vi "encodeStream.vi"(8 "error in (no error)":errorcluster, 11 "tBSONJavaScriptWithScope in":refnum<class "tBSONJavaScriptWithScope.lvclass">) -> (0 "error out":errorcluster, 2 "Byte Array":u8[](array[numeric]), 3 "tBSONJavaScriptWithScope out":refnum<class "tBSONJavaScriptWithScope.lvclass">)   [LabVIEW 2013, in "BSON.lvlib" / "tBSONJavaScriptWithScope.lvclass"]
uses:
  tBSONJavaScriptWithScope.lvclass
  tBSONElement/getName.vi
  tBSONJavaScript/getScript.vi
  getScope.vi
  tBSONDocument/tBSONDocument.lvclass
  BSON.lvlib
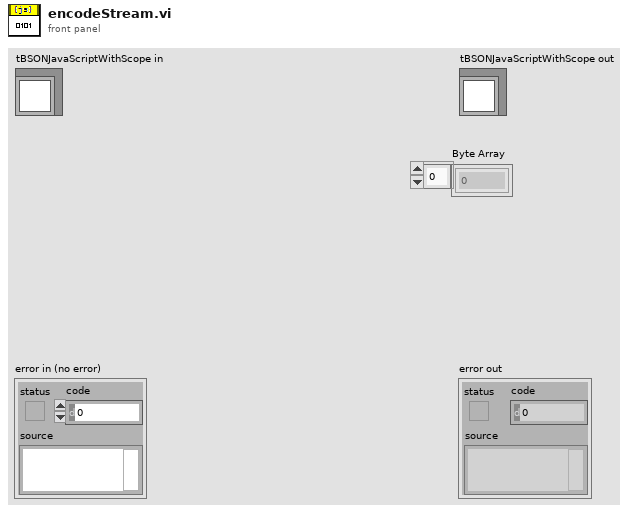
[diagram p1: front panel]
types:
  T1 = typedef "BSON.lvlib/tBSONElement.lvclass/type.ctl" = u8
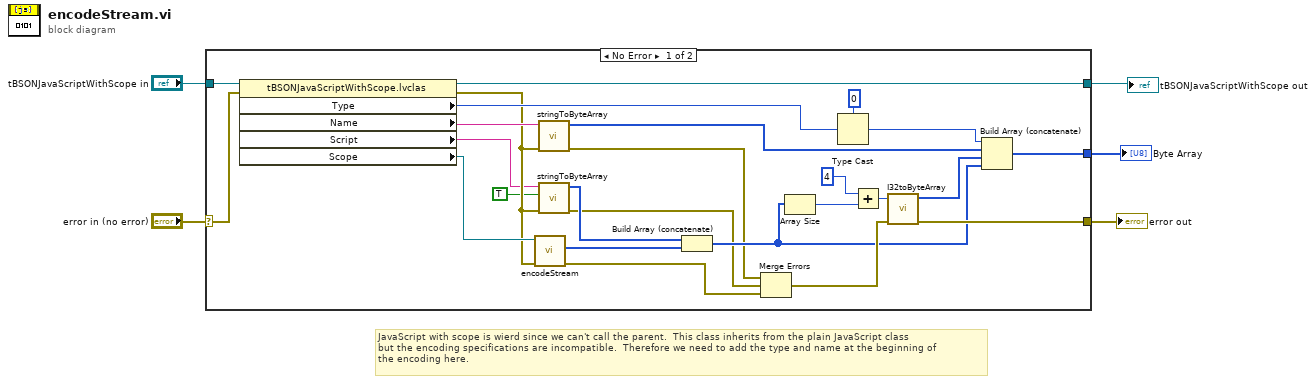
[diagram p0: block diagram]
diagram:
  # "JavaScript with scope is wierd since we can't call the parent.  This class inherits from the plain JavaScript class\nbut the encoding specifications are incompatible.  Therefore we need to add the type and name at the beginning of\nthe encoding here."
  n1 = case shown="No Error" "error in (no error)" {
    selector: "error in (no error)" -> [w29 w31]
    tunnel: "tBSONJavaScriptWithScope in" -> [w30 w32]
    tunnel: [w17 w32] -> w1
    tunnel: [w21 w31] -> w3
    tunnel: [w28 _] -> w2
    frame No Error {
      n2 = property class="tBSONJavaScriptWithScope.lvclas"(reference=w30, error in=w29) -> (reference out=w17:refnum<class "tBSONJavaScriptWithScope.lvclass">, error out=w10:errorcluster, "Type"=w15:T1, "Name"=w13:string, "Script"=w9:string, "Scope"=w26:refnum<class "tBSONDocument.lvclass">)
      n3 = call "encodeStream.vi"("error in (no error)"=w10, "tBSONDocument in"=w26) -> ("error out"=w27:errorcluster, "Byte Data"=w20:u8[])  [unwired: 7 in, 1 out]
      n4 = call "stringToByteArray.vi"("error in (no error)"=w10, "String"=w13) -> ("error out"=w12:errorcluster, "byte array"=w11:u8[])  [unwired: 8 in]
      n5 = call "stringToByteArray.vi"("error in (no error)"=w10, "Prepend Size"=TRUE, "String"=w9) -> ("error out"=w7:errorcluster, "byte array"=w8:u8[])  [unwired: 7 in]
      n6 = Build Array (concatenate)(w8, w20) -> (w18:u8[])
      n7 = Merge Errors(w12, w7, w27) -> (w23:errorcluster)
      n8 = Array Size(array=w18) -> (size(s)=w19:i32)
      n9 = Type Cast(type=u8 0, x=w15) -> (*(type *) &x=w14:u8)
      n10 = Add(x=4, y=w19) -> (x+y=w24:i32)
      n11 = call "I32toByteArray.vi"("error in (no error)"=w23, "I32"=w24) -> ("error out"=w21:errorcluster, "LittleEndianByteArray"=w22:u8[])  [unwired: 8 in]
      n12 = Build Array (concatenate)(w14, w11, w22, w18) -> (w28:u8[])
    }
    frame Error {
    }
  }
  "error out" <- w3
  "tBSONJavaScriptWithScope out" <- w1
  "Byte Array" <- w2
